vi "UHR-Fleezers Control (host) - 11.9.vi"() -> ()   [LabVIEW 2014] (continued)
                n3330 = Build Array (concatenate)(w5188, w5175) -> (w5187:dbl[])
                n3331 = Select(t=w5175, s=w5133, f=w5187) -> (s? t:f=w5162:dbl[])
                n3332 = feedback-in #40(w5162) -> ()
                n3333 = Divide(x=w5202, y=w5203) -> (x/y=w5205:dbl)
                n3334 = Multiply(x=w5205, y=100.0) -> (x*y=w5204:dbl)
                n3335 = Build Array(w5162, w5153) -> (→"Saved APD":dbl[][])
                n3336 = Array Size(array=w5162) -> (size(s)=w5180:i32)
                n3337 = Unbundle By Name(w5182) -> ("Y"=w5186:dbl[])
                n3338 = Subtract(x=w5180, y="N pts to average") -> (x-y=w5156:i32)
                n3339 = Multiply(x="N pts to average", y=u16 2) -> (x*y=w5157:u16)
                n3340 = Subtract(x=w5180, y=w5157) -> (x-y=w5155:i32)
                n3341 = feedback #41(w5186) -> (w5185:dbl[])
                n3342 = Build Array (concatenate)(w5185, w5186) -> (w5184:dbl[])
                n3343 = Select(t=w5186, s=w5133, f=w5184) -> (s? t:f=w5183:dbl[])
                "Trap Delta Graph" <- w5183
                n3344 = feedback-in #41(w5183) -> ()
                n3345 = Array Subset(array=w5162, index=w5156, length="N pts to average") -> (w5179:dbl[])
                n3346 = Array Subset(array=w5162, index=w5155, length="N pts to average") -> (w5178:dbl[])
                n3347 = Array Subset(array=w5153, index=w5156, length="N pts to average") -> (w5159:dbl[])
                n3348 = Array Subset(array=w5153, index=w5155, length="N pts to average") -> (w5158:dbl[])
                n3349 = Index Array(array=w5136, index=0) -> (element=w5134:waveform(dbl))
                n3350 = call-poly <vilib>:"Mean.vi"("X"=w5179) -> ("mean"=w5177:dbl)  [unwired: 1 out]
                n3351 = call-poly <vilib>:"Mean.vi"("X"=w5159) -> ("mean"=w5152:dbl)  [unwired: 1 out]
                n3352 = call-poly <vilib>:"Mean.vi"("X"=w5178) -> ("mean"=w5176:dbl)  [unwired: 1 out]
                n3353 = call-poly <vilib>:"Mean.vi"("X"=w5158) -> ("mean"=w5151:dbl)  [unwired: 1 out]
                n3354 = Unbundle By Name(w5134) -> ("Y"=w5131:dbl[])
                n3355 = Subtract(x=w5152, y=w5151) -> (x-y=w5143:dbl)
                "Delta Fl. 2" <- w5143
                n3356 = Subtract(x=w5177, y=w5176) -> (x-y=w5174:dbl)
                "Delta Fl. 1" <- w5174
                n3357 = Initialize Array(w5174, 1 ("dimension size")) -> (w5171:dbl[])
                n3358 = Initialize Array(w5143, 1 ("dimension size")) -> (w5148:dbl[])
                n3359 = feedback #42(w5171) -> (w5172:dbl[])
                n3360 = Build Array (concatenate)(w5172, w5171) -> (w5170:dbl[])
                n3361 = feedback #43(w5148) -> (w5149:dbl[])
                n3362 = Build Array (concatenate)(w5149, w5148) -> (w5147:dbl[])
                n3363 = feedback #44(w5131) -> (w5130:dbl[])
                n3364 = Build Array (concatenate)(w5130, w5131) -> (w5132:dbl[])
                n3365 = Select(t=w5131, s=w5133, f=w5132) -> (s? t:f=w5129:dbl[])
                "Saved trap pos" <- w5129
                n3366 = feedback-in #44(w5129) -> ()
                n3367 = Select(t=w5171, s=w5133, f=w5170) -> (s? t:f=w5146:dbl[])
                n3368 = feedback-in #42(w5146) -> ()
                n3369 = Select(t=w5148, s=w5133, f=w5147) -> (s? t:f=w5145:dbl[])
                n3370 = feedback-in #43(w5145) -> ()
                n3371 = Build Array(w5146, w5145) -> (→"Save APD Deriv":dbl[][])
              }
            }
            "Progress" <- w5112
            "Progress 2" <- w5112
          }
        }
      }
    }
    n3372 = Bundle By Name(cluster=w3707, "Green FB Ch 0"=w3706, "Green FB Ch 1"=w3705) -> (w3685:T48)
    "Green FB Signals (V)" <- w3685
    n3373 = Unbundle By Name(w3685) -> ("Green FB Ch 2"=→"Green FB Plot":dbl)
    n3374 = local read "wait to reset values"() -> (w3774:bool)
    n3375 = Not(x=w3772) -> (.not. x?=w3775:bool)
    n3376 = And(x=w3775, y=w3774) -> (x .and. y?=w3776:bool)
    n3377 = case "Part of MCL raster scanning: returns to initial positions after scan done" shown="True" w3776 {
      tunnel: w3494 -> [w4647 w4654]
      tunnel: [w4647 w4653] -> w3778
      tunnel: w3493 -> [w4646 w4652]
      tunnel: [w4646 w4651] -> w3773
      frame False {
      }
      frame True {
        w4662 = 10.0 ("y")
        w4661 = 32767.0 ("y")
        # "to return scan values\nafter a synchronous \nAOM scan"
        n3378 = local read "AO2"() -> (w4655:dbl)
        n3379 = local read "AO1"() -> (w4656:dbl)
        n3380 = local write "wait to reset values"(FALSE ("wait to reset values")) -> ()
        n3381 = Multiply(x=w4656, y=w4661) -> (x*y=w4658:dbl)
        n3382 = Multiply(x=w4655, y=w4661) -> (x*y=w4660:dbl)
        n3383 = Divide(x=w4658, y=w4662) -> (x/y=w4657:dbl)
        n3384 = Divide(x=w4660, y=w4662) -> (x/y=w4659:dbl)
        n3385 = To Word Integer(number=w4657) -> (16bit integer=w4663:i16)
        n3386 = To Word Integer(number=w4659) -> (16bit integer=w4664:i16)
        n3387 = local read "Total Counts (ticks)"() -> (w4648:u32)
        n3388 = xnode "Read/Write Control"("FPGA VI Reference In"=w4654, "error in"=w4652, "AO1"=w4663, "AO2"=w4664, "MCL count"=w4648) -> ("FPGA VI Reference Out"=w4653:T19, "error out"=w4651:errorcluster)
        n3389 = local read "Scan Range (V)\n(of steps)"() -> (w4649:dbl)
        n3390 = property on="Scan Range (V)\n(of steps)" class="DigNum (strict)"("Val(Sgnl)"=w4649) -> ()  [unwired: 2 in, 2 out]
      }
    }
    n3391 = node-c288() -> ()  [unwired: 2 out]
  }
  n3392 = VISA Close(VISA resource name=w101, error in (no error)=w100) -> (error out=w148:errorcluster)
  n3393 = call <vilib>:"Simple Error Handler.vi"("error in (no error)"=w148) -> ()  [unwired: 1 in, 8 out]
  n3394 = node-c288(w107) -> ()  [unwired: 1 out]
  n3395 = node-c288(w192) -> ()  [unwired: 1 out]
  n3396 = flat-sequence {
    tunnel: w284 -> [w5249]
    tunnel: w286 -> [w5250]
    tunnel: [w5248] -> w265
    tunnel: [w5247] -> w264
    tunnel: w248 -> [_]
    tunnel: w200 -> [_]
    tunnel: w113 -> [_]
    tunnel: w265 -> [w5251]
    tunnel: w264 -> [w5252]
    frame #0 {
      w5246 = FALSE ("AI to FIFO")
      n3397 = xnode "Read/Write Control"("FPGA VI Reference In"=w5250, "error in"=w5249, "AI to FIFO"=w5246, "APD to FIFO"=w5246) -> ("FPGA VI Reference Out"=w5248:T19, "error out"=w5247:errorcluster)
    }
    frame #1 {
      n3398 = xnode "Close FPGA VI Reference"("FPGA VI Reference In"=w5251, "error in"=w5252) -> ("error out"=→"error out":errorcluster)
    }
  }
  "Grn enabl" <- FALSE
